vi "HandleSetTemp.vi"(8 "error in (no error)":errorcluster, 11 "S4GUI in":refnum<class "S4GUI.lvclass">) -> (0 "error out":errorcluster, 3 "S4GUI out":refnum<class "S4GUI.lvclass">)   [LabVIEW 2018, in "S4GUI.lvclass"]
uses:
  S4GUI.lvclass
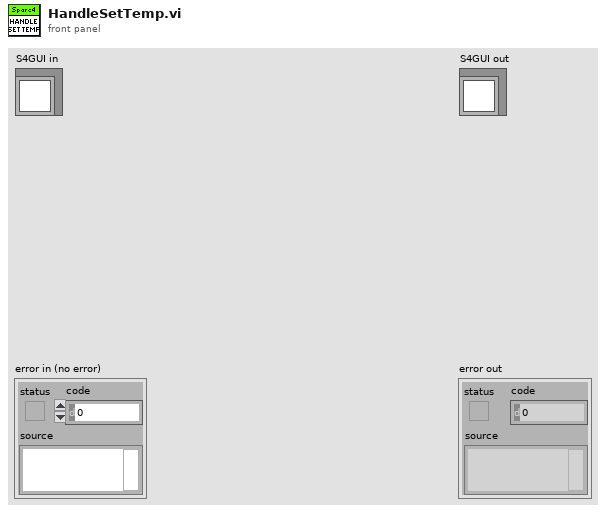
[diagram p1: front panel]
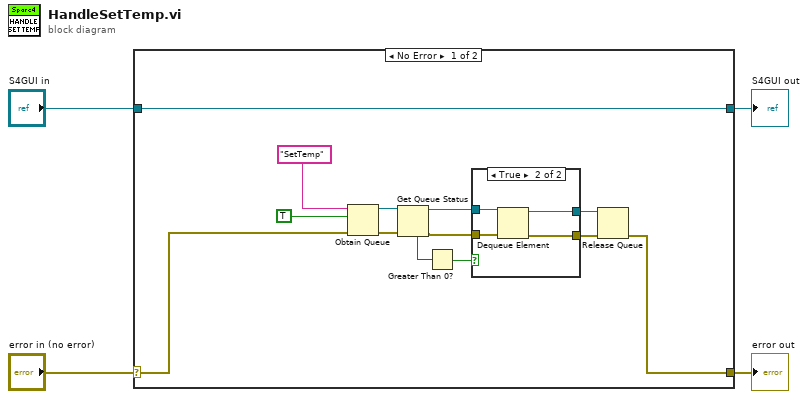
[diagram p0: block diagram]
diagram:
  n1 = case shown="No Error" "error in (no error)" {
    selector: "error in (no error)" -> [w7 w25]
    tunnel: [w6 w25] -> w3
    tunnel: [w17 w24] -> w1
    tunnel: "S4GUI in" -> [w17 w24]
    frame No Error {
      n2 = Obtain Queue(name (unnamed)="SetTemp", element data type=TRUE, error in (no error)=w7) -> (queue out=w14:refnum<queue>, error out=w15:errorcluster)  [unwired: 2 in, 1 out]
      n3 = Get Queue Status(queue=w14, error in (no error)=w15) -> (queue out=w11:refnum<queue>, error out=w10:errorcluster, # elements in queue=w13:i32)  [unwired: 1 in, 5 out]
      n4 = Greater Than 0?(x=w13) -> (x > 0?=w12:bool)
      n5 = case shown="True" w12 {
        tunnel: w11 -> [w19 w22]
        tunnel: w10 -> [w18 w23]
        tunnel: [w19 w21] -> w9
        tunnel: [w18 w20] -> w8
        frame False {
        }
        frame True {
          n6 = Dequeue Element(queue=w22, error in (no error)=w23) -> (queue out=w21:refnum<queue>, error out=w20:errorcluster)  [unwired: 1 in, 2 out]
        }
      }
      n7 = Release Queue(queue=w9, error in (no error)=w8) -> (error out=w6:errorcluster)  [unwired: 1 in, 2 out]
    }
    frame Error {
    }
  }
  "error out" <- w3
  "S4GUI out" <- w1
